vi "RenderRobotPose.vi"(0 "Robot X (in)":dbl, 1 "Robot Width (in)":dbl=30.0 format="%#_13g", 2 "Robot Length (in)":dbl=30.0 format="%#_13g", 3 "Buffer Time (min)":dbl=5.0 format="%#_13g", 5 "Robot Y (in)":dbl, 9 "Robot Heading (deg)":dbl, 11 "Turret Heading (deg)":dbl, 12 "Robot Enabled":bool, 14 "Reset":bool) -> (6 "Robot Pose":cluster{dbl[], dbl[]}[](graph))   [LabVIEW 2020]
doc: "This VI takes the robot pose information as input and renders a plot to display it. At this time, only square robot dimensions are supported."
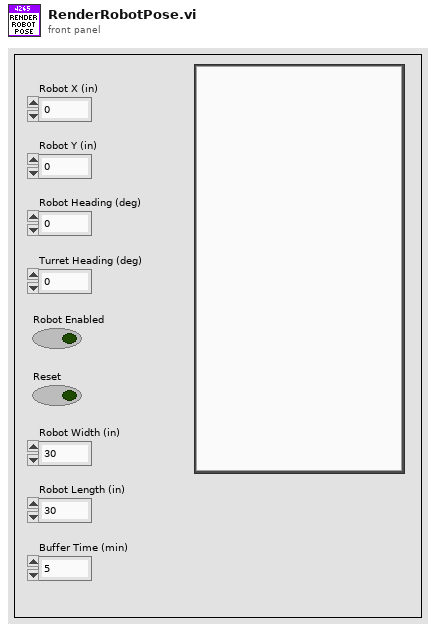
[diagram p1: front panel]
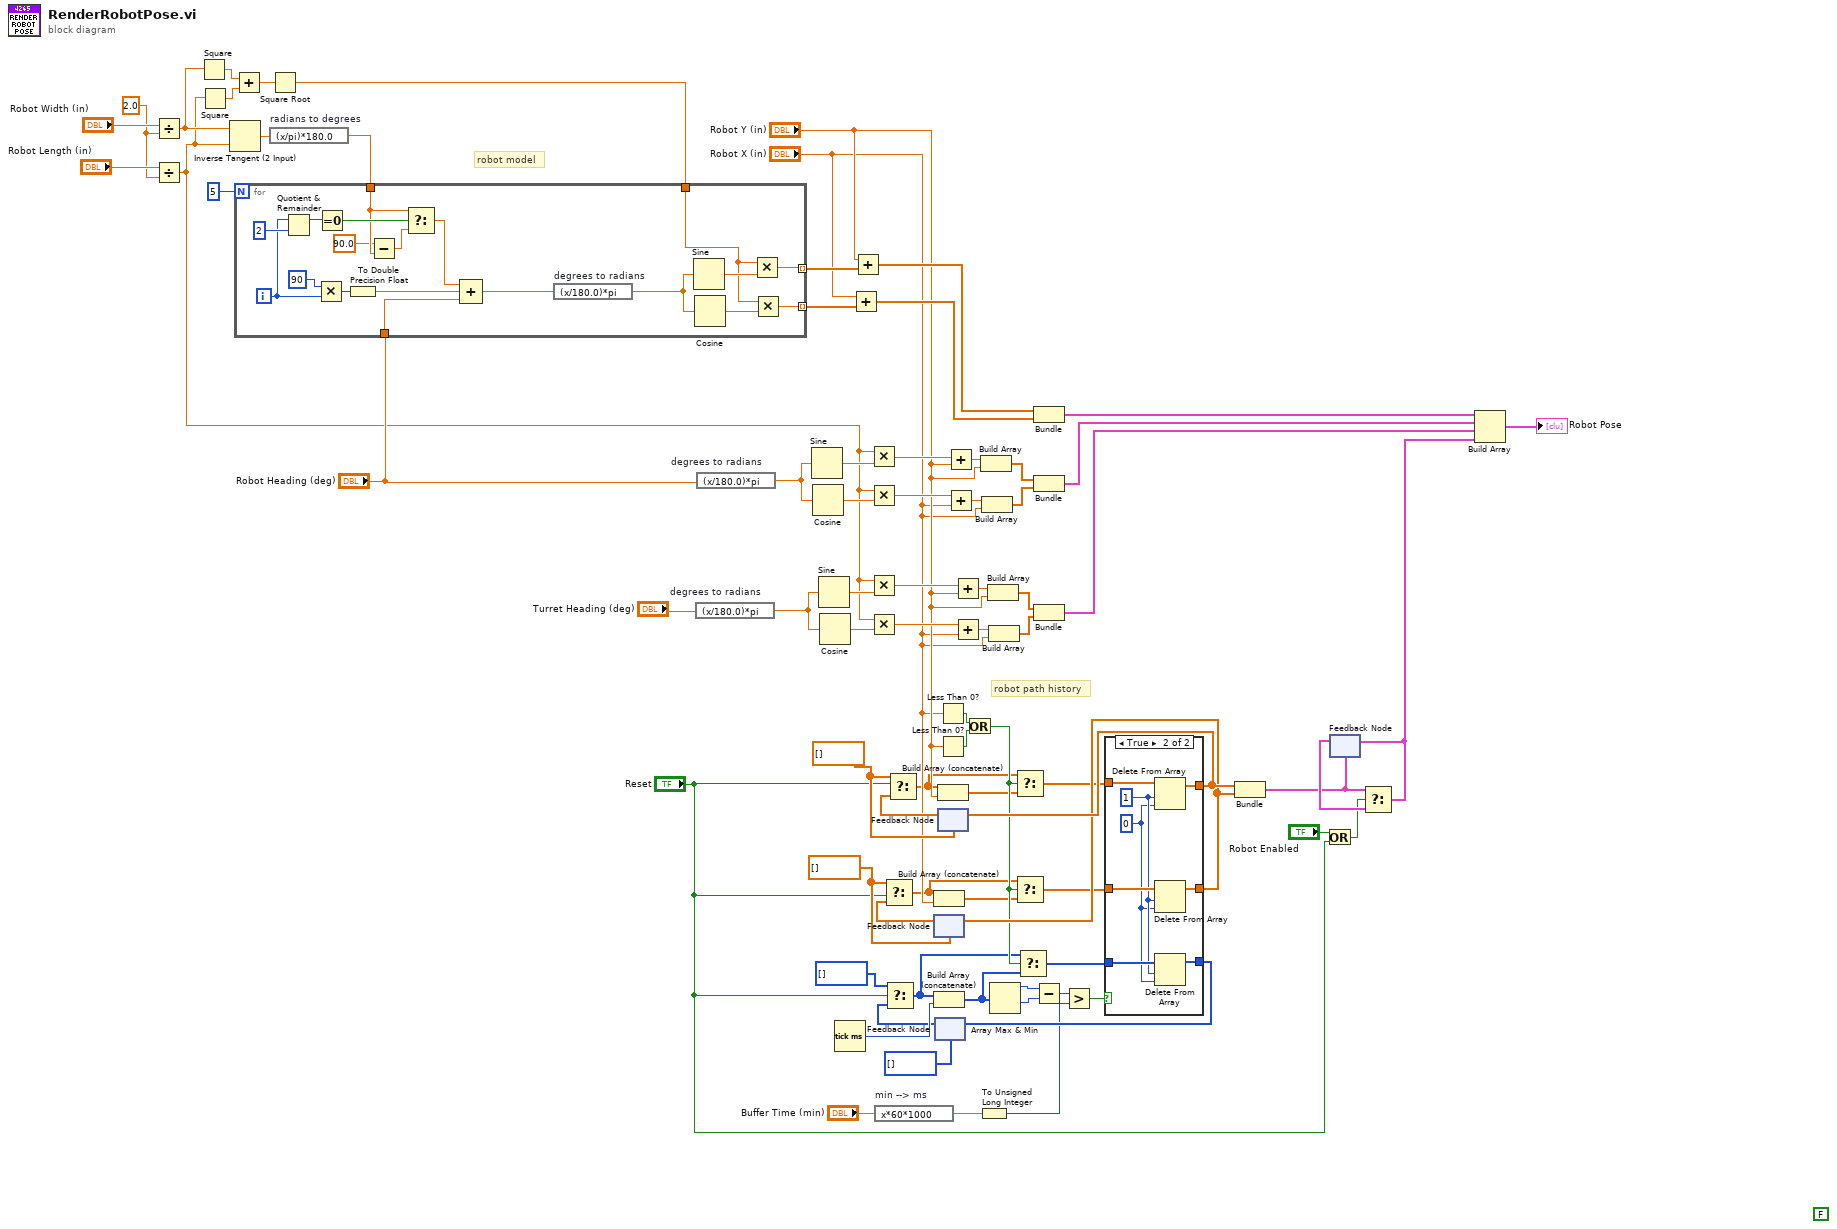
[diagram p0: block diagram]
diagram:
  w9 = 2.0
  (unwired) FALSE
  w28 = dbl[] [] ("t")
  w27 = dbl[] [] ("t")
  # "robot model"
  # "robot path history"
  n1 = Divide(x="Robot Width (in)", y=w9) -> (x/y=w6:dbl)
  n2 = Divide(x="Robot Length (in)", y=w9) -> (x/y=w5:dbl)
  n3 = Square(x=w6) -> (x^2=w3:dbl)
  n4 = Square(x=w5) -> (x^2=w4:dbl)
  n5 = Inverse Tangent (2 Input)(1:w5, 2:w6) -> (0:w8:dbl)
  n6 = Add(x=w3, y=w4) -> (x+y=w2:dbl)
  n7 = Square Root(x=w2) -> (sqrt(x)=w1:dbl)
  n8 = expression code="(x/pi)*180.0" "radians to degrees"(w8) -> (w7:dbl)
  n9 = for {
    N: 5 -> [_]
    tunnel: [w94] -> w77 mode=indexing
    tunnel: [w93] -> w76 mode=indexing
    tunnel: "Robot Heading (deg)" -> [w88]
    tunnel: w7 -> [w84]
    tunnel: w1 -> [w79]
    i -> [w80]
    n10 = Quotient & Remainder(x=w80, y=2) -> (x-y*floor(x/y)=w86:i32)  [unwired: 1 out]
    n11 = Multiply(x=90, y=w80) -> (x*y=w91:i32)
    n12 = Equal To 0?(x=w86) -> (x = 0?=w85:bool)
    n13 = To Double Precision Float(number=w91) -> (double precision float=w90:dbl)
    n14 = Subtract(x=90.0, y=w84) -> (x-y=w83:dbl)
    n15 = Select(t=w84, s=w85, f=w83) -> (s? t:f=w81:dbl)
    n16 = Compound Arithmetic op=ADD(w81, w90, w88) -> (w89:dbl)
    n17 = expression code="(x/180.0)*pi" "degrees to radians"(w89) -> (w96:dbl)
    n18 = Sine(x=w96) -> (sin(x)=w95:dbl)
    n19 = Cosine(x=w96) -> (cos(x)=w97:dbl)
    n20 = Multiply(x=w79, y=w95) -> (x*y=w93:dbl)
    n21 = Multiply(x=w79, y=w97) -> (x*y=w94:dbl)
  }
  n22 = expression code="(x/180.0)*pi" "degrees to radians"("Turret Heading (deg)") -> (w53:dbl)
  n23 = expression code="(x/180.0)*pi" "degrees to radians"("Robot Heading (deg)") -> (w42:dbl)
  n24 = Sine(x=w42) -> (sin(x)=w41:dbl)
  n25 = Cosine(x=w42) -> (cos(x)=w40:dbl)
  n26 = Sine(x=w53) -> (sin(x)=w52:dbl)
  n27 = Cosine(x=w53) -> (cos(x)=w51:dbl)
  n28 = Tick Count (ms)() -> (millisecond timer value=w60:u32)
  n29 = Add(x="Robot X (in)", y=w77) -> (x+y=w74:dbl[])
  n30 = Add(x="Robot Y (in)", y=w76) -> (x+y=w73:dbl[])
  n31 = Multiply(x=w5, y=w41) -> (x*y=w39:dbl)
  n32 = Multiply(x=w5, y=w40) -> (x*y=w38:dbl)
  n33 = Multiply(x=w5, y=w52) -> (x*y=w50:dbl)
  n34 = Multiply(x=w5, y=w51) -> (x*y=w49:dbl)
  n35 = expression code="x*60*1000" "min --> ms"("Buffer Time (min)") -> (w65:dbl)
  n36 = feedback #1(w27) -> (w56:dbl[])
  n37 = Select(t=w27, s="Reset", f=w56) -> (s? t:f=w16:dbl[])
  n38 = Build Array (concatenate)(w16, "Robot X (in)") -> (w17:dbl[])
  n39 = feedback #2(u32[] []) -> (w58:u32[])
  n40 = Select(t=u32[] [], s="Reset", f=w58) -> (s? t:f=w21:u32[])
  n41 = Build Array (concatenate)(w21, w60) -> (w20:u32[])
  n42 = Less Than 0?(x="Robot X (in)") -> (x < 0?=w24:bool)
  n43 = Less Than 0?(x="Robot Y (in)") -> (x < 0?=w25:bool)
  n44 = feedback #3(w28) -> (w59:dbl[])
  n45 = Select(t=w28, s="Reset", f=w59) -> (s? t:f=w18:dbl[])
  n46 = Build Array (concatenate)(w18, "Robot Y (in)") -> (w19:dbl[])
  n47 = Add(x=w39, y="Robot Y (in)") -> (x+y=w37:dbl)
  n48 = Add(x=w38, y="Robot X (in)") -> (x+y=w36:dbl)
  n49 = Add(x=w50, y="Robot Y (in)") -> (x+y=w48:dbl)
  n50 = Add(x=w49, y="Robot X (in)") -> (x+y=w47:dbl)
  n51 = Or(x=w24, y=w25) -> (x .or. y?=w23:bool)
  n52 = To Unsigned Long Integer(number=w65) -> (unsigned 32bit integer=w66:u32)
  n53 = Build Array(w37, "Robot Y (in)") -> (w35:dbl[])
  n54 = Build Array(w36, "Robot X (in)") -> (w34:dbl[])
  n55 = Build Array(w48, "Robot Y (in)") -> (w46:dbl[])
  n56 = Build Array(w47, "Robot X (in)") -> (w45:dbl[])
  n57 = Array Max & Min(array=w20) -> (max value=w62:u32, min value=w63:u32)  [unwired: 2 out]
  n58 = Select(t=w18, s=w23, f=w19) -> (s? t:f=w30:dbl[])
  n59 = Select(t=w16, s=w23, f=w17) -> (s? t:f=w29:dbl[])
  n60 = Select(t=w21, s=w23, f=w20) -> (s? t:f=w22:u32[])
  n61 = Bundle(w73, w74) -> (w44:cluster{dbl[], dbl[]})  [unwired: 1 in]
  n62 = Bundle(w35, w34) -> (w43:cluster{dbl[], dbl[]})  [unwired: 1 in]
  n63 = Bundle(w46, w45) -> (w54:cluster{dbl[], dbl[]})  [unwired: 1 in]
  n64 = Subtract(x=w62, y=w63) -> (x-y=w64:u32)
  n65 = Greater?(x=w64, y=w66) -> (0:w68:bool)
  n66 = case shown="True" w68 {
    tunnel: w22 -> [w98 w106]
    tunnel: w29 -> [w99 w107]
    tunnel: w30 -> [w100 w108]
    tunnel: [w100 w103] -> w71
    tunnel: [w99 w102] -> w70
    tunnel: [w98 w101] -> w69
    frame False {
    }
    frame True {
      w104 = 0 ("index")
      w105 = 1 ("length")
      n67 = Delete From Array(array=w108, length=w105, index=w104) -> (array with subset deleted=w103:dbl[])  [unwired: 1 out]
      n68 = Delete From Array(array=w107, length=w105, index=w104) -> (array with subset deleted=w102:dbl[])  [unwired: 1 out]
      n69 = Delete From Array(array=w106, length=w105, index=w104) -> (array with subset deleted=w101:u32[])  [unwired: 1 out]
    }
  }
  n70 = feedback-in #1(w70) -> ()
  n71 = feedback-in #2(w69) -> ()
  n72 = feedback-in #3(w71) -> ()
  n73 = Bundle("t"=w71, "t"=w70) -> (w33:cluster{"t":dbl[], "t":dbl[]})  [unwired: 1 in]
  n74 = Or(x="Robot Enabled", y="Reset") -> (x .or. y?=w13:bool)
  n75 = feedback #4(w33) -> (w72:cluster{"t":dbl[], "t":dbl[]})
  n76 = Select(t=w33, s=w13, f=w72) -> (s? t:f=w32:cluster{"t":dbl[], "t":dbl[]})
  n77 = feedback-in #4(w32) -> ()
  n78 = Build Array(w44, w43, w54, w32) -> (→"Robot Pose":cluster{"t":dbl[], "t":dbl[]}[])
